vi "Measure Peak.vi"(8 "error in (no error)":errorcluster, 11 "VISA resource name":refnum<visa-resource-name>) -> (0 "error out":errorcluster, 1 "Min Peak Current":dbl format="%_5g", 2 "Max Peak Current":dbl format="%_6f", 3 "VISA resource name out":refnum<visa-resource-name>, 4 "Min Peak Voltage":dbl format="%_6f", 5 "Max Peak Voltage":dbl format="%_6f")   [LabVIEW 2019, in "BK Precision 8500B Series.lvlib"]
doc: "Measures the Max/Min Peak Voltage, and Max/Min Peak Current."
uses:
  <instrlib>/BK Precision 8500B Series/BK Precision 8500B Series.lvlib
panel:
  # "V"
  # "V"
  # "A"
  # "A"
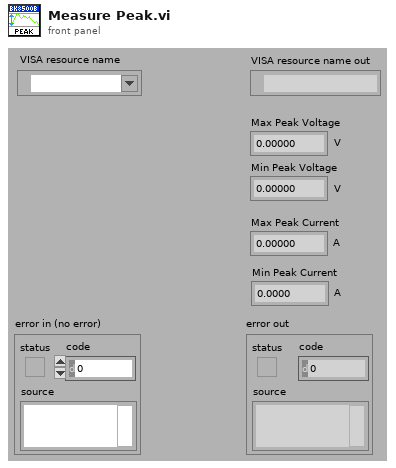
[diagram p1: front panel]
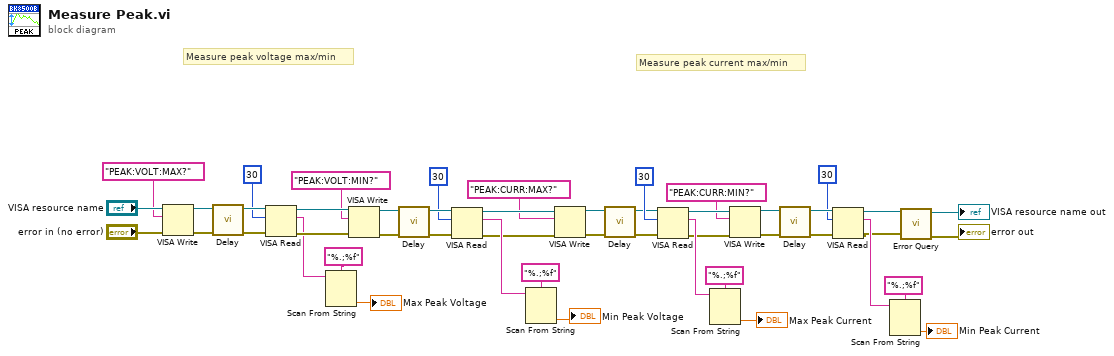
[diagram p0: block diagram]
diagram:
  # "Measure peak current max/min"
  # "Measure peak voltage max/min"
  n1 = VISA Write(VISA resource name="VISA resource name", write buffer="PEAK:VOLT:MAX?", error in (no error)="error in (no error)") -> (VISA resource name out=w45:refnum<visa-resource-name>, error out=w43:errorcluster)  [unwired: 1 out]
  n2 = call <instrlib>:"Delay.vi"("error in (no error)"=w43, "VISA resource name"=w45) -> ("error out"=w42:errorcluster, "VISA resource name out"=w44:refnum<visa-resource-name>)  [unwired: 8 in]
  n3 = VISA Read(VISA resource name=w44, byte count=30, error in (no error)=w42) -> (VISA resource name out=w41:refnum<visa-resource-name>, read buffer=w32:string, error out=w40:errorcluster)  [unwired: 1 out]
  n4 = Scan From String(format string="%.;%f", input string=w32) -> (output 1=→"Max Peak Voltage":dbl)  [unwired: 3 in, 3 out]
  n5 = VISA Write(VISA resource name=w41, write buffer="PEAK:VOLT:MIN?", error in (no error)=w40) -> (VISA resource name out=w39:refnum<visa-resource-name>, error out=w38:errorcluster)  [unwired: 1 out]
  n6 = call <instrlib>:"Delay.vi"("error in (no error)"=w38, "VISA resource name"=w39) -> ("error out"=w36:errorcluster, "VISA resource name out"=w37:refnum<visa-resource-name>)  [unwired: 8 in]
  n7 = VISA Read(VISA resource name=w37, byte count=30, error in (no error)=w36) -> (VISA resource name out=w28:refnum<visa-resource-name>, read buffer=w30:string, error out=w27:errorcluster)  [unwired: 1 out]
  n8 = Scan From String(format string="%.;%f", input string=w30) -> (output 1=→"Min Peak Voltage":dbl)  [unwired: 3 in, 3 out]
  n9 = VISA Write(VISA resource name=w28, write buffer="PEAK:CURR:MAX?", error in (no error)=w27) -> (VISA resource name out=w25:refnum<visa-resource-name>, error out=w24:errorcluster)  [unwired: 1 out]
  n10 = call <instrlib>:"Delay.vi"("error in (no error)"=w24, "VISA resource name"=w25) -> ("error out"=w21:errorcluster, "VISA resource name out"=w22:refnum<visa-resource-name>)  [unwired: 8 in]
  n11 = VISA Read(VISA resource name=w22, byte count=30, error in (no error)=w21) -> (VISA resource name out=w11:refnum<visa-resource-name>, read buffer=w20:string, error out=w10:errorcluster)  [unwired: 1 out]
  n12 = Scan From String(format string="%.;%f", input string=w20) -> (output 1=→"Max Peak Current":dbl)  [unwired: 3 in, 3 out]
  n13 = VISA Write(VISA resource name=w11, write buffer="PEAK:CURR:MIN?", error in (no error)=w10) -> (VISA resource name out=w18:refnum<visa-resource-name>, error out=w16:errorcluster)  [unwired: 1 out]
  n14 = call <instrlib>:"Delay.vi"("error in (no error)"=w16, "VISA resource name"=w18) -> ("error out"=w15:errorcluster, "VISA resource name out"=w17:refnum<visa-resource-name>)  [unwired: 8 in]
  n15 = VISA Read(VISA resource name=w17, byte count=30, error in (no error)=w15) -> (VISA resource name out=w3:refnum<visa-resource-name>, read buffer=w14:string, error out=w2:errorcluster)  [unwired: 1 out]
  n16 = Scan From String(format string="%.;%f", input string=w14) -> (output 1=→"Min Peak Current":dbl)  [unwired: 3 in, 3 out]
  n17 = call <instrlib>:"Error Query.vi"("error in (no error)"=w2, "VISA resource name"=w3) -> ("error out"=→"error out":errorcluster, "VISA resource name out"=→"VISA resource name out":refnum<visa-resource-name>)  [unwired: 6 in, 2 out]
